vi "Test.vi"() -> ()   [LabVIEW 2020, in "Sprachverwaltung.lvlib"]
uses:
  Sprachverwaltung.lvlib
panel:
  in  "Registerkartenelement":enum32{"Seite 1", "Seite 2"}(tab)
  in  "Cluster":T1
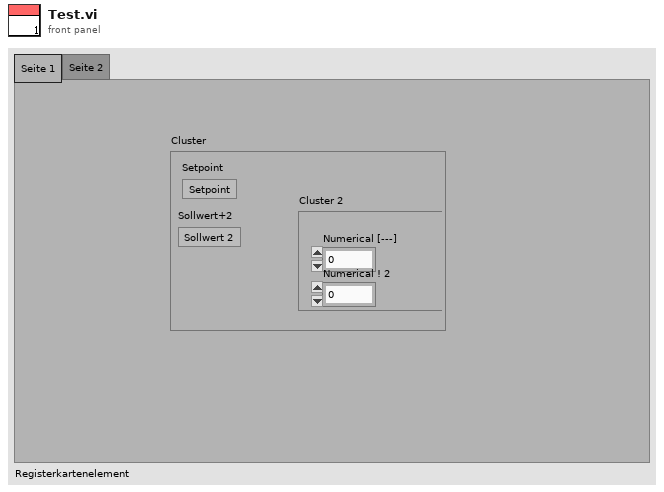
[diagram p1: front panel]
types:
  T1 = cluster{"Sollwert":bool, "Cluster 2":cluster{"Numerisch":dbl, "Numerisch 2":dbl}, "Sollwert 2":bool}
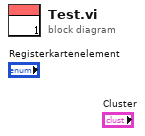
[diagram p0: block diagram]
diagram:
